vi "Get Full Force Test Settings.vi"(11 "Model in":refnum<class "Model.lvclass">) -> (2 "Full Force Test Settings":T1 {"SAA Force Set Points"."Axial Force" format="%.4f"; "SAA Force Set Points"."Lateral Force" format="%.4f"; "Sample Time (s)" format="%.4f"; "Process Time (s)" format="%.4f"; "DAA Force Set Points"."Axial Force" format="%.4f"; "DAA Force Set Points"."Lateral Force" format="%.4f"; "Force Tolerance (N)" format="%.4f"}, 3 "Model out":refnum<class "Model.lvclass">)   [LabVIEW 2016, in "Model.lvclass"]
uses:
  Model.lvclass
  Typedefs/FullForceScanSettings.ctl
  Typedefs/ForcePair.ctl
  Model.lvclass/Model.ctl
  Typedefs/FAMT Typedefs.lvlib
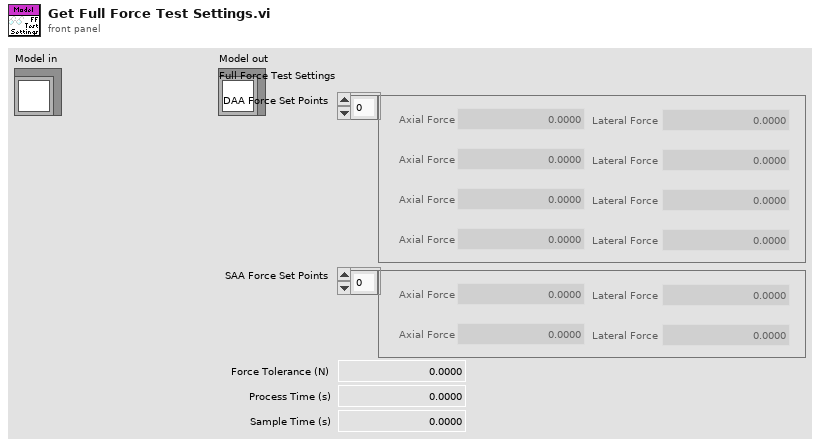
[diagram p1: front panel]
types:
  T1 = typedef "FAMT Typedefs.lvlib/FullForceScanSettings.ctl" = cluster{"Force Tolerance (N)":dbl, "DAA Force Set Points":T2[], "Process Time (s)":dbl, "Sample Time (s)":dbl, "SAA Force Set Points":T2[]}
  T2 = typedef "FAMT Typedefs.lvlib/ForcePair.ctl" = cluster{"Axial Force":dbl, "Lateral Force":dbl}
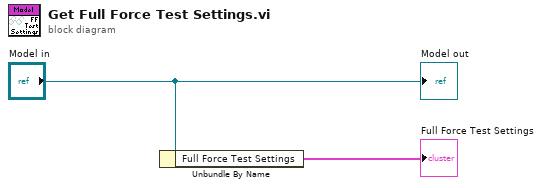
[diagram p0: block diagram]
diagram:
  n1 = Unbundle By Name("Model in") -> ("Full Force Test Settings"=→"Full Force Test Settings":T1)
  "Model out" <- "Model in"
